vi "Example - Queue-based operations.vi"() -> ()   [LabVIEW 2020, in "wamplv.lvlib"]
uses:
  wamplv.lvlib
  WAMP Client/WAMP Client.lvclass
  86c89e9c-a710-438b-81a6-9e903d6b3f4b.vi
  7b7e4b67-f0c8-4bef-b1e5-f1b849c8dc8e.vi
  b30a270a-9252-4db6-9284-e54c33467919.vi
panel:
  in  "Unregister RPC":bool caption="Publish Topic"
  in  "Endpoint return value":string="Hello, world!"
  in  "Register RPC":bool caption="Publish Topic"
  out "Error URI":string
  out "Callee Error?":bool
  out "Call Result ArgumentKw":string
  out "Call Result Arguments":string
  in  "Call Arguments":string[](array[string])
  in  "Call URI":string="test.endpoint"
  in  "Call":bool caption="Publish Topic"
  in  "Unsubscribe":bool caption="Publish Topic"
  out "Topic:":string
  out "ArgumentKw Payload":string
  out "Arguments Payload":string
  out "Event received on:":string
  in  "Publish Argument Payload":string[](array[string])
  in  "Subscription URI":string="test.topic"
  in  "Subscribe":bool caption="Publish Topic"
  in  "Disconnect":bool caption="Publish Topic"
  in  "Realm":string="default_realm"
  in  "Topic URI":string="test.topic"
  in  "Publish":bool caption="Publish Topic"
  in  "Router Address":string="ws://localhost:8080/"
  # "Endpoint name: test.endpoint"
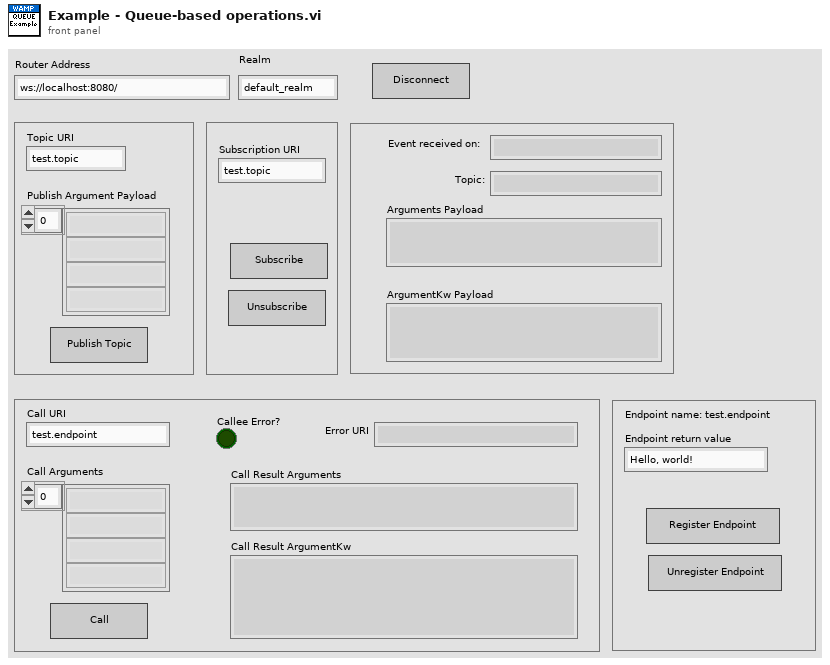
[diagram p1: front panel]
types:
  T1 = typedef "wamplv.lvlib/WAMP Client.lvclass/WAMP error.ctl" = cluster{"Details":string, "ArgumentKw Payload":string, "Error?":bool, "Error URI":string, "Arguments Payload":string}
  T2 = typedef "wamplv.lvlib/WAMP Client.lvclass/INVOCATION payload.ctl" = cluster{"Arguments":string, "ArgumentKw":string, "Procedure URI":string, "Details":string, "Registration ID":u64, "Invocation Request ID":refnum<class "Invocation Request ID.lvclass">}
  T3 = typedef "wamplv.lvlib/WAMP Client.lvclass/EVENT payload.ctl" = cluster{"Arguments Payload":string, "ArgumentKw Payload":string, "Topic":string}
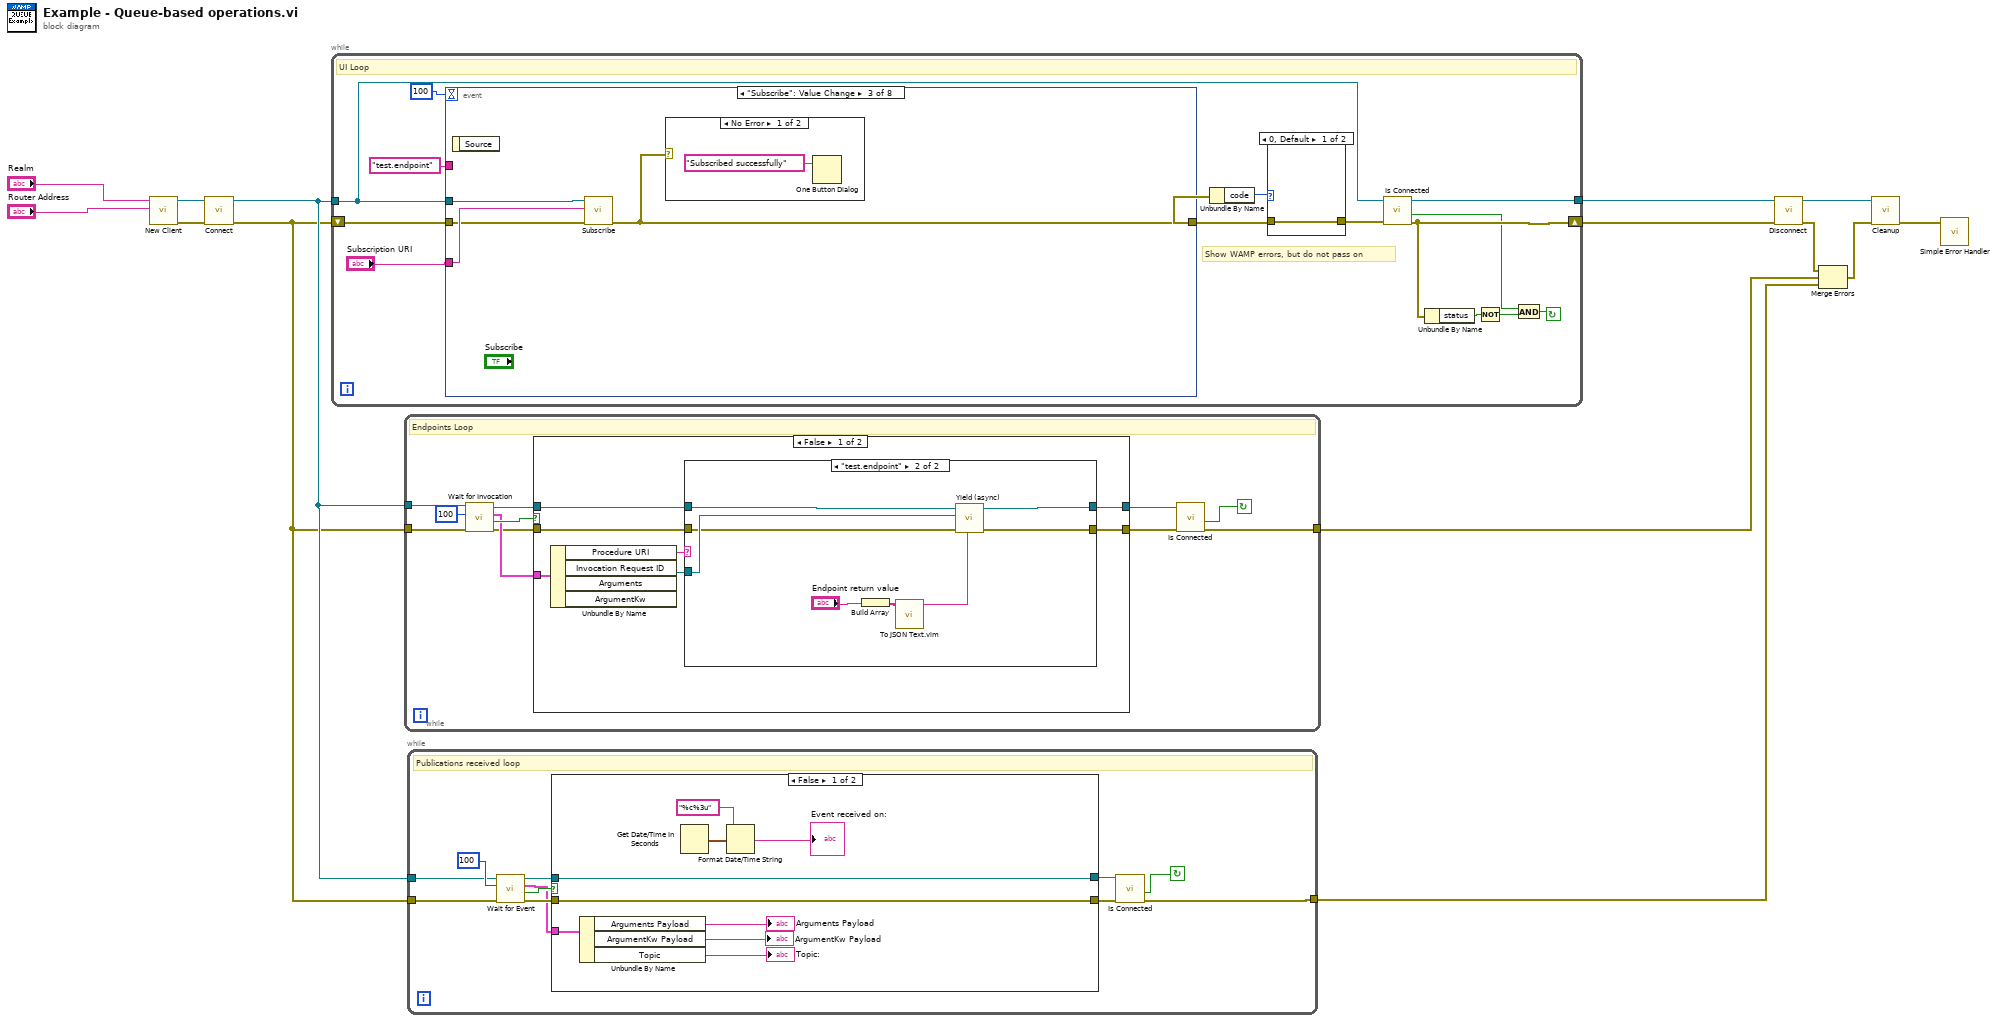
[diagram p0: block diagram]
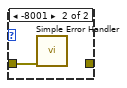
[diagram p5: hidden frame]
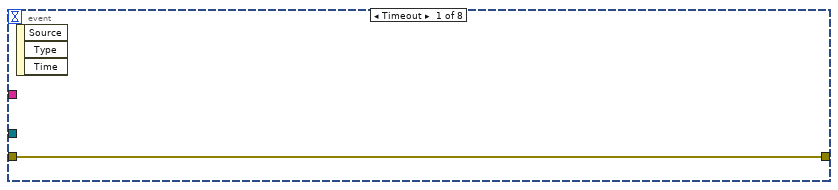
[diagram p6: hidden frame]
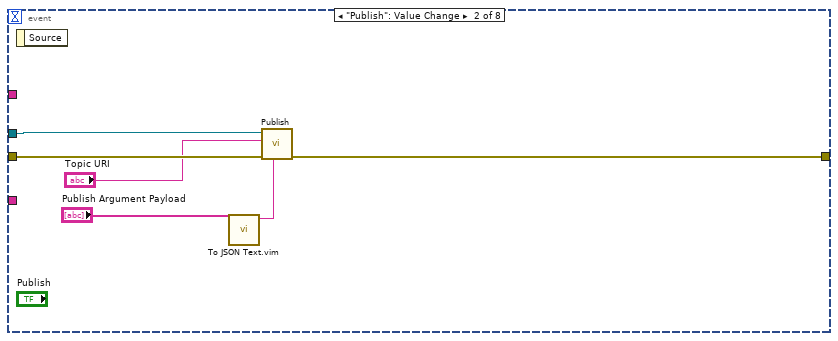
[diagram p7: hidden frame]
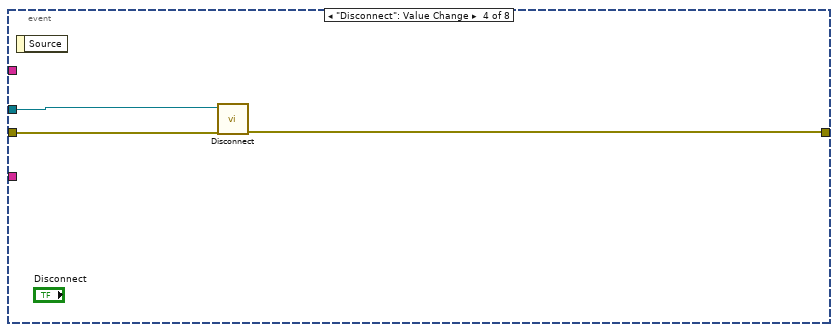
[diagram p9: hidden frame]
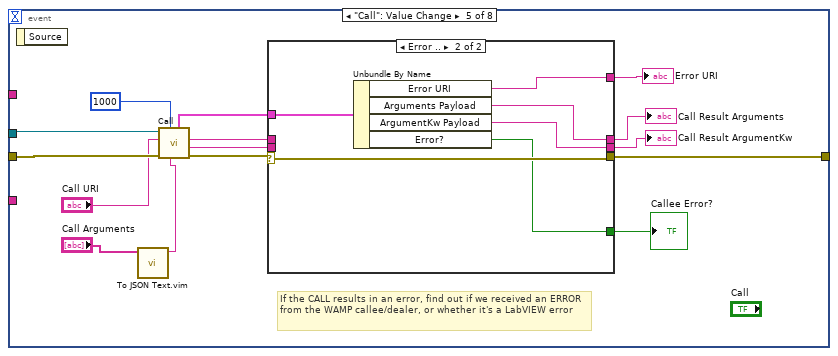
[diagram p10: hidden frame]
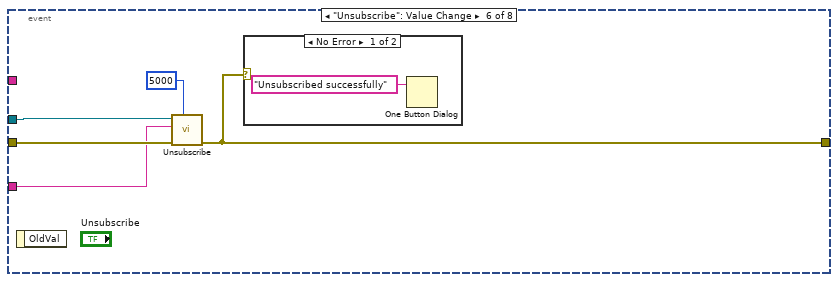
[diagram p12: hidden frame]
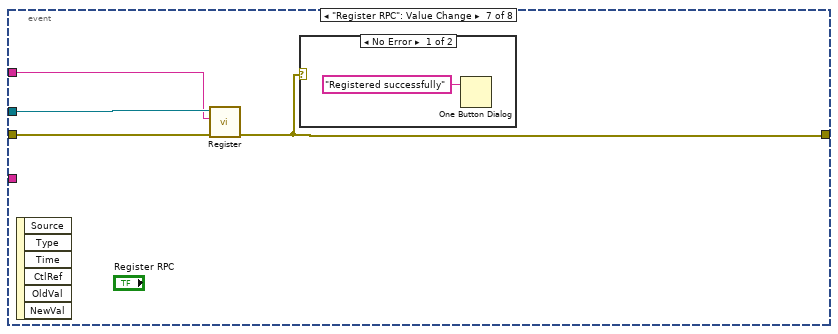
[diagram p14: hidden frame]
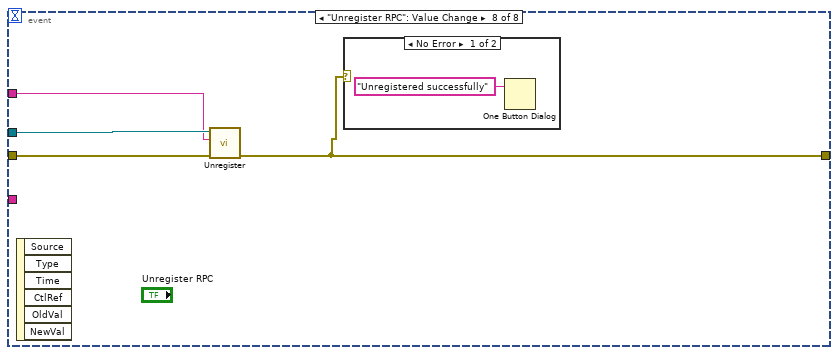
[diagram p16: hidden frame]
diagram:
  n1 = call "New Client.vi"("Address"="Router Address", "Realm"="Realm") -> ("error out"=w4:errorcluster, "WAMP client out"=w12:refnum<class "WAMP Client.lvclass">)  [unwired: 8 in]
  n2 = call "Connect.vi"("error in"=w4, "WAMP Client in"=w12) -> ("error out"=w3:errorcluster, "WAMP Client out"=w6:refnum<class "WAMP Client.lvclass">)  [unwired: 8 in]
  n3 = while {
    tunnel: w6 -> [w26]
    shift-right: [w18] -> w2
    shift-left: w3 -> [w28]
    tunnel: [w25] -> w5
    stop <- w19 continue-if-true
    # "Show WAMP errors, but do not pass on"
    # "UI Loop"
    n4 = event shown="[2] \"Subscribe\": Value Change" {
      selector: _ -> [_ _ _ _ _ _ _ _]
      dyn-events: _ -> [_ _ _ _ _ _ _ _]
      timeout: 100 -> [_ _ _ _ _ _ _ _]
      tunnel: w26 -> [_ w37 w41 w45 w60 w73 w79 w84]
      tunnel: w28 -> [w31 w36 w39 w44 w59 w74 w78 w83]
      tunnel: [w31 w35 w38 w43 w56 w70 w76 w81] -> w21
      tunnel: "Subscription URI" -> [_ _ w40 _ _ w72 _ _]
      tunnel: "test.endpoint" ("Procedure URI") -> [_ _ _ _ _ _ w77 w82]
      event Timeout {
        n5 = event-data() -> ()  [unwired: 1 in, 3 out]
      }
      event "Publish": Value Change {
        n6 = event-data() -> ()  [unwired: 1 in, 1 out]
        n7 = call "To JSON Text.vim"("Anything"="Publish Argument Payload") -> ("<JSON>"=w32:string)  [unwired: 9 in, 1 out]
        n8 = call "Publish.vi"("Arguments"=w32, "Error in"=w36, "Topic"="Topic URI", "WAMP Client in"=w37) -> ("Error out"=w35:errorcluster)  [unwired: 5 in, 2 out]
      }
      event "Subscribe": Value Change {
        n9 = event-data() -> ()  [unwired: 1 in, 1 out]
        n10 = call-dynamic "Subscribe.vi"("error in (no error)"=w39, "Topic"=w40, "WAMP Client in"=w41) -> ("error out"=w38:errorcluster)  [unwired: 5 in, 3 out]
        n11 = case shown="No Error" w38 {
          frame No Error {
            n12 = One Button Dialog(message="Subscribed successfully") -> ()  [unwired: 1 in, 1 out]
          }
          frame Error {
          }
        }
      }
      event "Disconnect": Value Change {
        n13 = event-data() -> ()  [unwired: 1 in, 1 out]
        n14 = call-dynamic "Disconnect.vi"("error in"=w44, "WAMP Client in"=w45) -> ("error out"=w43:errorcluster)  [unwired: 8 in, 1 out]
      }
      event "Call": Value Change {
        # "If the CALL results in an error, find out if we received an ERROR from the WAMP callee/dealer, or whether it's a LabVIEW error"
        n15 = event-data() -> ()  [unwired: 1 in, 1 out]
        n16 = call "To JSON Text.vim"("Anything"="Call Arguments") -> ("<JSON>"=w46:string)  [unwired: 9 in, 1 out]
        n17 = call-dynamic "Call.vi"("Arguments"=w46, "Timeout (ms)"=1000 ("Numeric"), "Error in"=w59, "Topic URI"="Call URI", "WAMP Client in"=w60) -> ("Error out"=w57:errorcluster, "ArgumentKw Payload"=w53:string, "Arguments Payload"=w54:string, "WAMP Error"=w49:T1)  [unwired: 2 in, 1 out]
        n18 = case shown="Error .." w57 {
          selector: w57 -> [w63 w65]
          tunnel: [w63 w65] -> w56
          tunnel: [w62 w69] -> w55
          tunnel: w54 -> [w62 _]
          tunnel: w53 -> [w61 _]
          tunnel: [w61 w68] -> w52
          tunnel: [_ w66] -> w50
          tunnel: w49 -> [_ w67]
          tunnel: [_ w64] -> w48
          frame No Error {
          }
          frame Error {
            n19 = Unbundle By Name(w67) -> ("Error URI"=w66:string, "Arguments Payload"=w69:string, "ArgumentKw Payload"=w68:string, "Error?"=w64:bool)
          }
        }
        "Call Result Arguments" <- w55
        "Callee Error?" <- w48
        "Call Result ArgumentKw" <- w52
        "Error URI" <- w50
      }
      event "Unsubscribe": Value Change {
        n20 = event-data() -> ()  [unwired: 1 in, 1 out]
        n21 = call-dynamic "Unsubscribe.vi"("Time out (1000 ms)"=5000 ("Time out (ms)"), "error in (no error)"=w74, "Topic"=w72, "WAMP Client in"=w73) -> ("error out"=w70:errorcluster)  [unwired: 6 in, 1 out]
        n22 = case shown="No Error" w70 {
          frame No Error {
            n23 = One Button Dialog(message="Unsubscribed successfully") -> ()  [unwired: 1 in, 1 out]
          }
          frame Error {
          }
        }
      }
      event "Register RPC": Value Change {
        n24 = event-data() -> ()  [unwired: 1 in, 6 out]
        n25 = call-dynamic "Register.vi"("Error in"=w78, "Procedure URI"=w77, "WAMP Client in"=w79) -> ("Error out"=w76:errorcluster)  [unwired: 6 in, 2 out]
        n26 = case shown="No Error" w76 {
          frame No Error {
            n27 = One Button Dialog(message="Registered successfully") -> ()  [unwired: 1 in, 1 out]
          }
          frame Error {
          }
        }
      }
      event "Unregister RPC": Value Change {
        n28 = event-data() -> ()  [unwired: 1 in, 6 out]
        n29 = call-dynamic "Unregister.vi"("error in (no error)"=w83, "URI"=w82, "WAMP Client in"=w84) -> ("error out"=w81:errorcluster)  [unwired: 6 in, 2 out]
        n30 = case shown="No Error" w81 {
          frame No Error {
            n31 = One Button Dialog(message="Unregistered successfully") -> ()  [unwired: 1 in, 1 out]
          }
          frame Error {
          }
        }
      }
    }
    n32 = Unbundle By Name(w21) -> ("code"=w22:i32)
    n33 = case shown="0, Default" w22 {
      tunnel: w21 -> [w29 w30]
      tunnel: [w29 _] -> w20
      frame 0, Default {
      }
      frame -8001 {
        n34 = call <vilib>:"Simple Error Handler.vi"("error in (no error)"=w30) -> ()  [unwired: 4 in, 5 out]
      }
    }
    n35 = call "Is Connected.vi"("error in"=w20, "WAMP Client in"=w26) -> ("error out"=w18:errorcluster, "Is Connected?"=w15:bool, "WAMP Client out"=w25:refnum<class "WAMP Client.lvclass">)  [unwired: 7 in]
    n36 = Unbundle By Name(w18) -> ("status"=w17:bool)
    n37 = Not(x=w17) -> (.not. x?=w16:bool)
    n38 = And(x=w15, y=w16) -> (x .and. y?=w19:bool)
  }
  n39 = while {
    tunnel: w6 -> [w96]
    tunnel: w3 -> [w95]
    tunnel: [w86] -> w8
    stop <- w87 continue-if-true
    # "Endpoints Loop"
    n40 = call "Wait for Invocation.vi"("error in (no error)"=w95, "timeout in ms (-1)"=100, "WAMP Client in"=w96) -> ("error out"=w90:errorcluster, "timed out?"=w93:bool, "WAMP Invocation"=w91:T2, "WAMP Client out"=w92:refnum<class "WAMP Client.lvclass">)  [unwired: 5 in]
    n41 = case shown="False" w93 {
      tunnel: w92 -> [w101 w115]
      tunnel: w91 -> [w103 _]
      tunnel: w90 -> [w99 w114]
      tunnel: [w98 w114] -> w88
      tunnel: [w97 w115] -> w89
      frame False {
        n42 = Unbundle By Name(w103) -> ("Procedure URI"=w102:string, "Invocation Request ID"=w100:refnum<class "Invocation Request ID.lvclass">)  [unwired: 2 out]
        n43 = case shown="\"test.endpoint\"" w102 {
          tunnel: w101 -> [w105 w113]
          tunnel: w100 -> [_ w112]
          tunnel: w99 -> [w104 w111]
          tunnel: [w104 w110] -> w98
          tunnel: [w105 w109] -> w97
          frame Default {
          }
          frame "test.endpoint" {
            n44 = Build Array("Endpoint return value") -> (w107:string[])
            n45 = call "To JSON Text.vim"("Anything"=w107) -> ("<JSON>"=w106:string)  [unwired: 9 in, 1 out]
            n46 = call "Yield (async).vi"("Arguments"=w106, "error in (no error)"=w111, "Invocation Request"=w112, "WAMP Client in"=w113) -> ("error out"=w110:errorcluster, "WAMP Client out"=w109:refnum<class "WAMP Client.lvclass">)  [unwired: 6 in]
          }
        }
      }
      frame True {
      }
    }
    n47 = call "Is Connected.vi"("error in"=w88, "WAMP Client in"=w89) -> ("error out"=w86:errorcluster, "Is Connected?"=w87:bool)  [unwired: 7 in, 1 out]
  }
  n48 = while {
    tunnel: w6 -> [w125]
    tunnel: w3 -> [w124]
    tunnel: [w116] -> w7
    stop <- w117 continue-if-true
    # "Publications received loop"
    n49 = call "Wait for Event.vi"("error in (no error)"=w124, "timeout in ms (-1)"=100, "WAMP Client in"=w125) -> ("error out"=w121:errorcluster, "timed out?"=w123:bool, "WAMP Event"=w120:T3, "WAMP Client out"=w122:refnum<class "WAMP Client.lvclass">)  [unwired: 5 in]
    n50 = case shown="False" w123 {
      tunnel: w122 -> [w128 w136]
      tunnel: w121 -> [w127 w137]
      tunnel: w120 -> [w132 _]
      tunnel: [w128 w136] -> w119
      tunnel: [w127 w137] -> w118
      frame False {
        n51 = Unbundle By Name(w132) -> ("Arguments Payload"=→"Arguments Payload":string, "ArgumentKw Payload"=→"ArgumentKw Payload":string, "Topic"=→"Topic:":string)
        n52 = Get Date/Time In Seconds() -> (seconds since 1Jan1904=w134:timestamp)
        n53 = Format Date/Time String(time format string (%c)="%c%3u", seconds (now)=w134) -> (date/time string=→"Event received on:":string)  [unwired: 1 in]
      }
      frame True {
      }
    }
    n54 = call "Is Connected.vi"("error in"=w118, "WAMP Client in"=w119) -> ("error out"=w116:errorcluster, "Is Connected?"=w117:bool)  [unwired: 7 in, 1 out]
  }
  n55 = call-dynamic "Disconnect.vi"("error in"=w2, "WAMP Client in"=w5) -> ("error out"=w1:errorcluster, "WAMP Client out"=w11:refnum<class "WAMP Client.lvclass">)  [unwired: 8 in]
  n56 = Merge Errors(w1, w8, w7) -> (w10:errorcluster)
  n57 = call-dynamic "Cleanup.vi"("error in"=w10, "WAMP Client in"=w11) -> ("error out"=w9:errorcluster)  [unwired: 8 in, 1 out]
  n58 = call <vilib>:"Simple Error Handler.vi"("error in (no error)"=w9) -> ()  [unwired: 4 in, 5 out]
